vi "FrequencyResponse.vi"(10 "DAC Codes":u16[](array[numeric]), 11 "Sampling Frequency (Hz)":u64) -> (2 "Frequency Response":cluster{dbl[], dbl[]}, 3 "DC Offset":dbl)   [LabVIEW 2018]
uses:
  <vilib>/Analysis/2dsp.llb/Real FFT.vi
  <vilib>/Analysis/NI_AALPro.lvlib
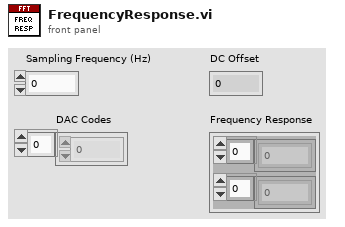
[diagram p1: front panel]
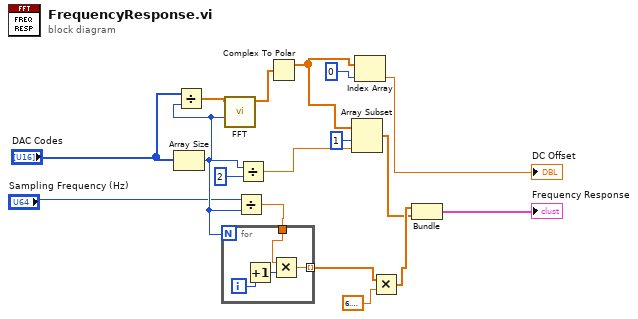
[diagram p0: block diagram]
diagram:
  n1 = Array Size(array="DAC Codes") -> (size(s)=w11:i32)
  n2 = Divide(x="DAC Codes", y=w11) -> (x/y=w1:dbl[])
  n3 = call-poly <vilib>:"FFT.vi"("FFT size"=w11, "X"=w1) -> ("FFT {X}"=w3:cdb[])  [unwired: 8 in, 1 out]
  n4 = Divide(x="Sampling Frequency (Hz)", y=w11) -> (x/y=w7:dbl)
  n5 = for {
    N: w11 -> [_]
    tunnel: w7 -> [w21]
    tunnel: [w19] -> w12 mode=indexing
    i -> [w20]
    n6 = Increment(x=w20) -> (x+1=w18:i32)
    n7 = Multiply(x=w21, y=w18) -> (x*y=w19:dbl)
  }
  n8 = Divide(x=w11, y=2) -> (x/y=w10:dbl)
  n9 = Complex To Polar(r * e^(i*theta)=w3) -> (r=w16:dbl[])  [unwired: 1 out]
  n10 = Array Subset(array=w16, index=1, length=w10) -> (w8:dbl[])
  n11 = Index Array(array=w16, index=0) -> (element=→"DC Offset":dbl)
  n12 = Multiply(x=w12, y=6.283185307179586) -> (x*y=w13:dbl[])
  n13 = Bundle(w13, w8) -> (→"Frequency Response":cluster{dbl[], dbl[]})  [unwired: 1 in]
